vi "Session Connect Write.vi"(8 "error in":errorcluster, 10 "Request Data":T1, 11 "Call ID in":T2) -> (0 "error out":errorcluster, 2 "Success":bool, 3 "Call ID":T2)   [LabVIEW 2019, in "Generated_client.lvlib"]
uses:
  Generated_client.lvlib
  9647bdd3-bda2-4565-bbb9-d670be58a455.vi
  <vilib>/gRPC/LabVIEW gRPC Library/Shared/grpcId.ctl
  <vilib>/gRPC/LabVIEW gRPC Library/grpc-lvsupport-release.lvlib
  RPC Messages/w4lvgrpc_ToServer_payload/w4lvgrpc_ToServer_payload.lvclass
  RPC Messages/w4lvgrpc_ToServer.ctl
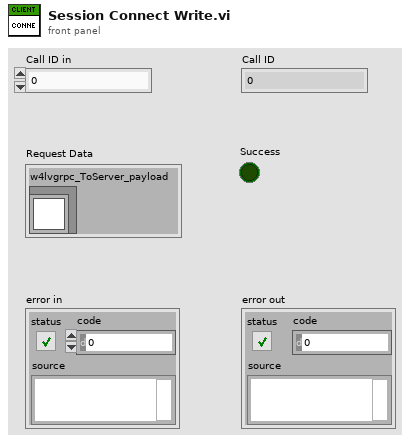
[diagram p1: front panel]
types:
  T1 = typedef "Generated_client.lvlib/w4lvgrpc_ToServer.ctl" = cluster{"w4lvgrpc_ToServer_payload":refnum<class "w4lvgrpc_ToServer_payload.lvclass">}
  T2 = typedef "grpc-lvsupport-release.lvlib/grpcId.ctl" = u64
  T3 = typedef "Generated_client.lvlib/w4lvgrpc_ToServer_Flat.ctl" = cluster{"w4lvgrpc_ToServer_payload_selected_index":i32, "msg_1":T4, "msg_2":T5, "msg_3":T6, "msg_4":T7, "msg_5":T8, "msg_6":T9, "msg_7":T10, "msg_8":T11, "msg_9":T12}
  T4 = typedef "Generated_client.lvlib/w4lvgrpc_Msg_ToServer_1_Flat.ctl" = cluster{"placeholder":string}
  T5 = typedef "Generated_client.lvlib/w4lvgrpc_Msg_ToServer_2_Flat.ctl" = cluster{"placeholder":string}
  T6 = typedef "Generated_client.lvlib/w4lvgrpc_Msg_ToServer_3_Flat.ctl" = cluster{"placeholder":string}
  T7 = typedef "Generated_client.lvlib/w4lvgrpc_Msg_ToServer_4_Flat.ctl" = cluster{"placeholder":string}
  T8 = typedef "Generated_client.lvlib/w4lvgrpc_Msg_ToServer_5_Flat.ctl" = cluster{"placeholder":string}
  T9 = typedef "Generated_client.lvlib/w4lvgrpc_Msg_ToServer_6_Flat.ctl" = cluster{"placeholder":string}
  T10 = typedef "Generated_client.lvlib/w4lvgrpc_Msg_ToServer_7_Flat.ctl" = cluster{"placeholder":string}
  T11 = typedef "Generated_client.lvlib/w4lvgrpc_Msg_ToServer_8_Flat.ctl" = cluster{"placeholder":string}
  T12 = typedef "Generated_client.lvlib/w4lvgrpc_Msg_ToServer_9_Flat.ctl" = cluster{"placeholder":string}
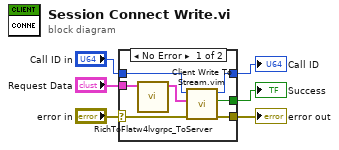
[diagram p0: block diagram]
diagram:
  n1 = case shown="No Error" "error in" {
    selector: "error in" -> [w13 w14]
    tunnel: [w12 w14] -> w5
    tunnel: "Call ID in" -> [w11 w15]
    tunnel: [w10 w15] -> w3
    tunnel: "Request Data" -> [w8 _]
    tunnel: [w9 _] -> w1
    frame No Error {
      n2 = call "RichToFlatw4lvgrpc_ToServer.vi"("InputCluster"=w8) -> ("OutputCluster"=w7:T3)  [unwired: 10 in]
      n3 = call "Client Write To Stream.vim"("error in"=w13, "Request Data"=w7, "Call ID in"=w11) -> ("error out"=w12:errorcluster, "Success"=w9:bool, "Call ID out"=w10:u64)  [unwired: 6 in]
    }
    frame Error {
    }
  }
  "error out" <- w5
  "Call ID" <- w3
  "Success" <- w1
